vi "Get Switching Info and Set Properties.vi"(7 "Close?":bool=TRUE, 8 "error in (no error)":errorcluster, 10 "Relays":refnum<class "Relay.lvclass">[](array[class]), 11 "SLSC Session In":T1) -> (0 "error out":errorcluster, 1 "property resources":string[](array[string]), 3 "SLSC Session Out":T1)   [LabVIEW 2015]
uses:
  SLSC Session/Typedefs/Session Handle.ctl
  SLSC Session/SLSC Session.lvclass
  Relay/Relay.lvclass
  Relay/Relay.lvclass/Relay.ctl
  Unique String Buffer/Unique String Buffer.lvclass
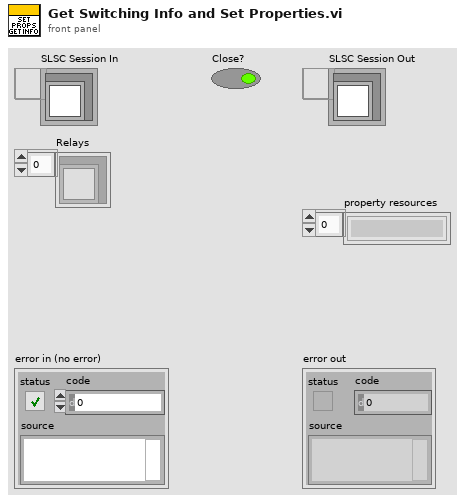
[diagram p1: front panel]
types:
  T1 = typedef "SLSC Switch.lvlib/SLSC Session.lvclass/Session Handle.ctl" = refnum<data-value>
  T2 = typedef "SLSC Switch.lvlib/Relay.lvclass/Property.ctl" = cluster{"resource name":string, "property":refnum<k21>}
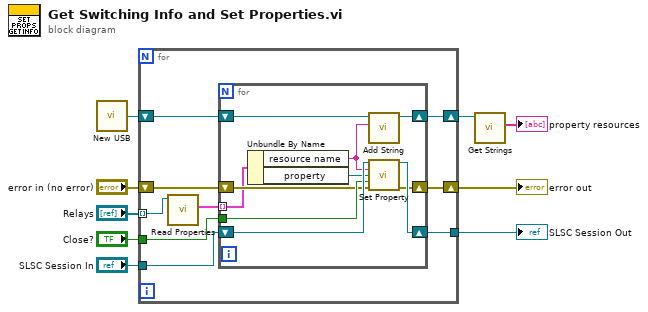
[diagram p0: block diagram]
diagram:
  n1 = call "New USB.vi"() -> ("Buffer out"=w5:refnum<class "Unique String Buffer.lvclass">)  [unwired: 2 in]
  n2 = for {
    tunnel: "Relays" -> [w10] mode=indexing
    tunnel: "SLSC Session In" -> [w18]
    tunnel: "Close?" -> [w17]
    tunnel: [w16] -> w4
    shift-right: [w12] -> w2
    shift-left: "error in (no error)" -> [w13]
    shift-right: [w14] -> w6
    shift-left: w5 -> [w15]
    n3 = call "Read Properties.vi"("Relay in"=w10) -> ("Properties"=w11:T2[])  [unwired: 8 in, 2 out]
    n4 = for {
      tunnel: w17 -> [w27]
      shift-right: [w26] -> w16
      shift-left: w18 -> [w28]
      shift-right: [w24] -> w14
      shift-left: w15 -> [w25]
      shift-right: [w22] -> w12
      shift-left: w13 -> [w23]
      tunnel: w11 -> [w21] mode=indexing
      n5 = Unbundle By Name(w21) -> ("resource name"=w20:string, "property"=w19:refnum<k21>)
      n6 = call "Add String.vi"("string"=w20, "Buffer in"=w25) -> ("Buffer out"=w24:refnum<class "Unique String Buffer.lvclass">)  [unwired: 8 in, 1 out]
      n7 = call "Set Property.vi"("Session Handle in"=w28, "resources"=w20, "property"=w19, "property value"=w27, "error in (no error)"=w23) -> ("Session Handle out"=w26:T1, "error out"=w22:errorcluster)  [unwired: 9 in]
    }
  }
  "SLSC Session Out" <- w4
  "error out" <- w2
  n8 = call "Get Strings.vi"("Buffer in"=w6) -> ("strings"=→"property resources":string[])  [unwired: 8 in, 2 out]
